vi "GUI Init - AIMV.vi"(8 "error in (no error)":errorcluster, 9 "Ch.names":string[](array[string]), 10 "Cluster":T2 {"Ch.value" min=-10.0 max=10.0 step=1.0 format="%.3g"}, 11 "GUI Refs":T1) -> (0 "error out":errorcluster, 2 "Data":dbl[](array[numeric]), 3 "reference out":refnum<vi>)   [LabVIEW 2017]
doc: "Initialize array's size and values for AIMV Array by reference"
uses:
  Controls/AIMV_GUI_Cluster.ctl
  Controls/GUI Referencies.ctl
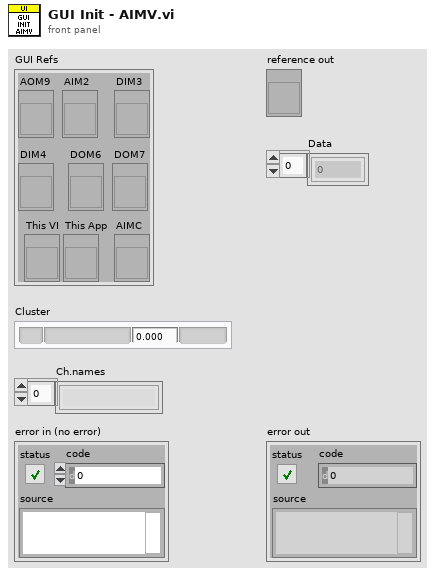
[diagram p1: front panel]
types:
  T1 = typedef "GUI Referencies.ctl" = cluster{"This VI":refnum<vi>, "This App":refnum<vi>, "DIM3":refnum<vi>, "DIM4":refnum<vi>, "DOM6":refnum<vi>, "DOM7":refnum<vi>, "AOM9":refnum<vi>, "AIM2":refnum<vi>, "AIMC":refnum<vi>}
  T2 = typedef "AIMV_GUI_Cluster.ctl" = cluster{"Ch.name":string, "Ch.value":dbl, "Ch.range":string, "Num":string}
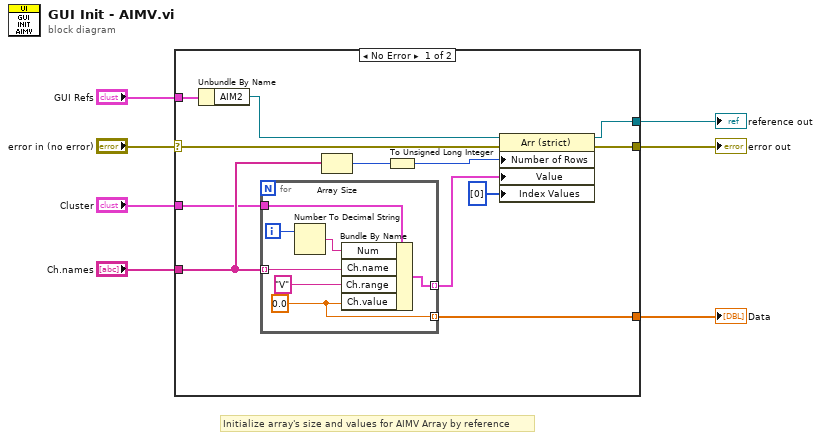
[diagram p0: block diagram]
diagram:
  # "Initialize array's size and values for AIMV Array by reference"
  n1 = case shown="No Error" "error in (no error)" {
    selector: "error in (no error)" -> [w13 w27]
    tunnel: [w12 w27] -> w6
    tunnel: "Ch.names" -> [w15 _]
    tunnel: "GUI Refs" -> [w10 _]
    tunnel: "Cluster" -> [w14 _]
    tunnel: [w11 _] -> w3
    tunnel: [w8 _] -> w1
    frame No Error {
      n2 = Unbundle By Name(w10) -> ("AIM2"=w9:refnum<vi>)
      n3 = for {
        tunnel: [w26] -> w11 mode=indexing
        tunnel: [w25] -> w19 mode=indexing
        tunnel: w15 -> [w23] mode=indexing
        tunnel: w14 -> [w22]
        i -> [w21]
        w26 = 0.0 ("Ch.value")
        n4 = Number To Decimal String(number=w21) -> (decimal integer string=w20:string)  [unwired: 1 in]
        n5 = Bundle By Name(cluster=w22, "Num"=w20, "Ch.name"=w23, "Ch.range"="V", "Ch.value"=w26) -> (w25:T2)
      }
      n6 = Array Size(array=w15) -> (size(s)=w17:i32)
      n7 = To Unsigned Long Integer(number=w17) -> (unsigned 32bit integer=w16:u32)
      n8 = property class="Arr (strict)"(reference=w9, error in=w13, "Number of Rows"=w16, "Value"=w19, "Index Values"=u32[] [0]) -> (reference out=w8:refnum<vi>, error out=w12:errorcluster)
    }
    frame Error {
    }
  }
  "error out" <- w6
  "Data" <- w3
  "reference out" <- w1
